vi "monitor_odczytZpc.vi"(11 "ramki jazdy 2":T1[](array[typedef]) {"type" items=["CAN Data", "CAN Remote"]; "identifier" format="%.0x"}) -> (0 "ramki jazdy out":T1[](array[typedef]) {"type" items=["CAN Data", "CAN Remote"]; "identifier" format="%.0x"}, 3 "Przestarza³a data":bool caption="Time has Elapsed")   [LabVIEW 2015]
uses:
  <vilib>/RioEmbeddedCAN/RioEmbeddedCAN.llb/CANFrameControl.ctl
  <vilib>/Utility/Variable/NI_VariableUtilities.lvlib
panel:
  in  "ramki jazdy zerowanie":T1[](array[typedef])=[{"identifier"=1, "extended?"=FALSE, "type"=0, "payload"=[1, 127, 255, 127, 255, 127, 255, 0]}, {"identifier"=2, "extended?"=FALSE, "type"=0, "payload"=[1, 127, 255, 127, 255, 127, 255, 0]}] {"type" items=["CAN Data", "CAN Remote"]; "identifier" format="%.0x"}
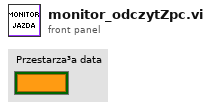
[diagram p1: front panel]
types:
  T1 = typedef "CANFrameControl.ctl" = cluster{"identifier":u32, "extended?":bool, "type":u8, "payload":u8[]}
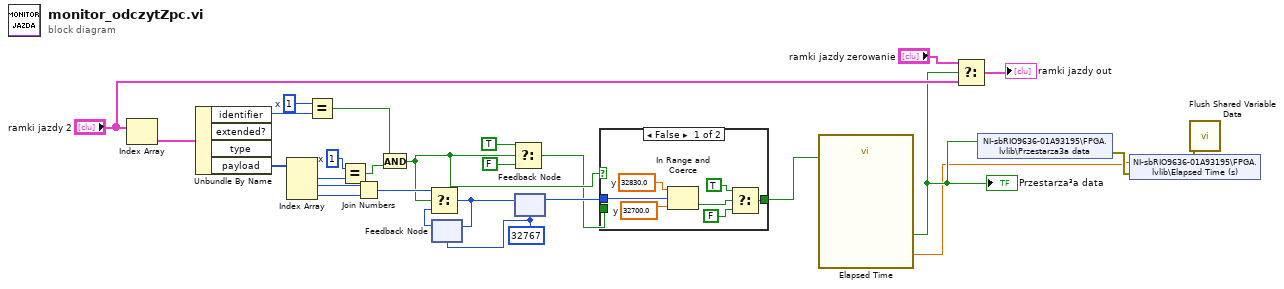
[diagram p0: block diagram]
diagram:
  w8 = u16 32767
  w22 = u8 1  # x
  w25 = u32 1  # x
  n1 = Index Array(array="ramki jazdy 2") -> (element=w27:T1)  [unwired: 1 in]
  n2 = Unbundle By Name(w27) -> ("identifier"=w26:u32, "payload"=w24:u8[])  [unwired: 2 out]
  n3 = Index Array(array=w24) -> (element #1=w23:u8, element #2=w21:u8, element #3=w20:u8)  [unwired: 3 in]
  n4 = Equal?(x=w25, y=w26) -> (x = y?=w19:bool)
  n5 = Equal?(x=w22, y=w23) -> (x = y?=w18:bool)
  n6 = Join Numbers(hi=w21, lo=w20) -> ((hi.lo)=w16:u16)
  n7 = And(x=w19, y=w18) -> (x .and. y?=w13:bool)
  n8 = feedback #1(w8) -> (w15:u16)
  n9 = Select(t=w16, s=w13, f=w15) -> (s? t:f=w9:u16)
  n10 = feedback-in #1(w9) -> ()
  n11 = Select(t=TRUE, s=w13, f=FALSE) -> (s? t:f=w12:bool)
  n12 = feedback #2(w8) -> (w17:u16)
  n13 = feedback-in #2(w9) -> ()
  n14 = case shown="False" w13 {
    tunnel: w17 -> [w32 _]
    tunnel: [w31 w35] -> w14
    tunnel: w12 -> [_ w35]
    frame False {
      w33 = 32830.0  # y
      w34 = 32700.0  # y
      n15 = In Range and Coerce(upper limit=w33, x=w32, lower limit=w34) -> (In Range?=w28:bool)  [unwired: 1 out]
      n16 = Select(t=TRUE, s=w28, f=FALSE) -> (s? t:f=w31:bool)
    }
    frame True {
    }
  }
  n17 = call "Elapsed Time"("Reset"=w14) -> ("Elapsed Time (s)"=w1:dbl, "Time has Elapsed"=w4:bool)  [unwired: 11 in, 6 out]
  "Przestarza³a data" <- w4
  n18 = Select(t="ramki jazdy zerowanie", s=w4, f="ramki jazdy 2") -> (s? t:f=→"ramki jazdy out":T1[])
  n19 = shared-variable "NI-sbRIO9636-01A93195\\FPGA.lvlib\\Przestarza3a data"(w4) -> (error out=w3:errorcluster)  [unwired: 1 in]
  n20 = shared-variable "NI-sbRIO9636-01A93195\\FPGA.lvlib\\Elapsed Time (s)"(w1, error in=w3) -> (error out=w2:errorcluster)
  n21 = call <vilib>:"Flush Shared Variable Data.vi"("error in (no error)"=w2) -> ()  [unwired: 10 in, 1 out]
